vi "LPT-LIBS-Spectra Acquire.vi"(8 "error in":errorcluster, 9 "Exposure time [ms]":dbl=50.0 format="%#.6g", 10 "LIBS Dark Array":dbl[](array[numeric])) -> (0 "error out":errorcluster, 1 "Removed background":dbl[](graph), 2 "Raw Data":dbl[](graph), 3 "Spectrum":cluster{dbl[], dbl[]}(graph))   [LabVIEW 2019]
uses:
  <vilib>/Analysis/NI_AAL_SigProc.lvlib
panel:
  in  "threshold":dbl format="%0.2f"
  out "Locations":dbl[](array[numeric])
  out "Amplitudes":dbl[](array[numeric])
  out "# found":i32
  in  "polynomial order":i32=3
  in  "baseline (0)":dbl
  in  "RCF radius (25)":i32=60
  out "Filtered Spectrum":cluster{"Wavelengths":dbl[], "Filtered X":dbl[]}(graph)
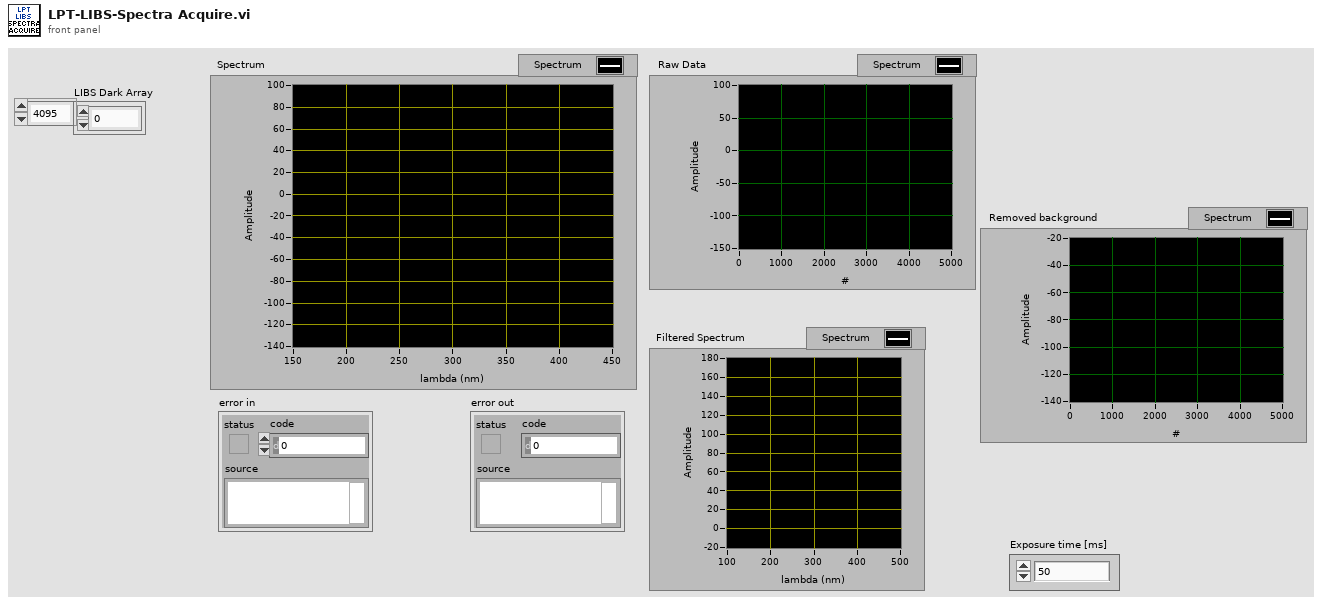
[diagram p1: front panel]
types:
  T1 = cluster{"Wavelength axis":dbl[], "Mean raw spectrum":dbl[]}
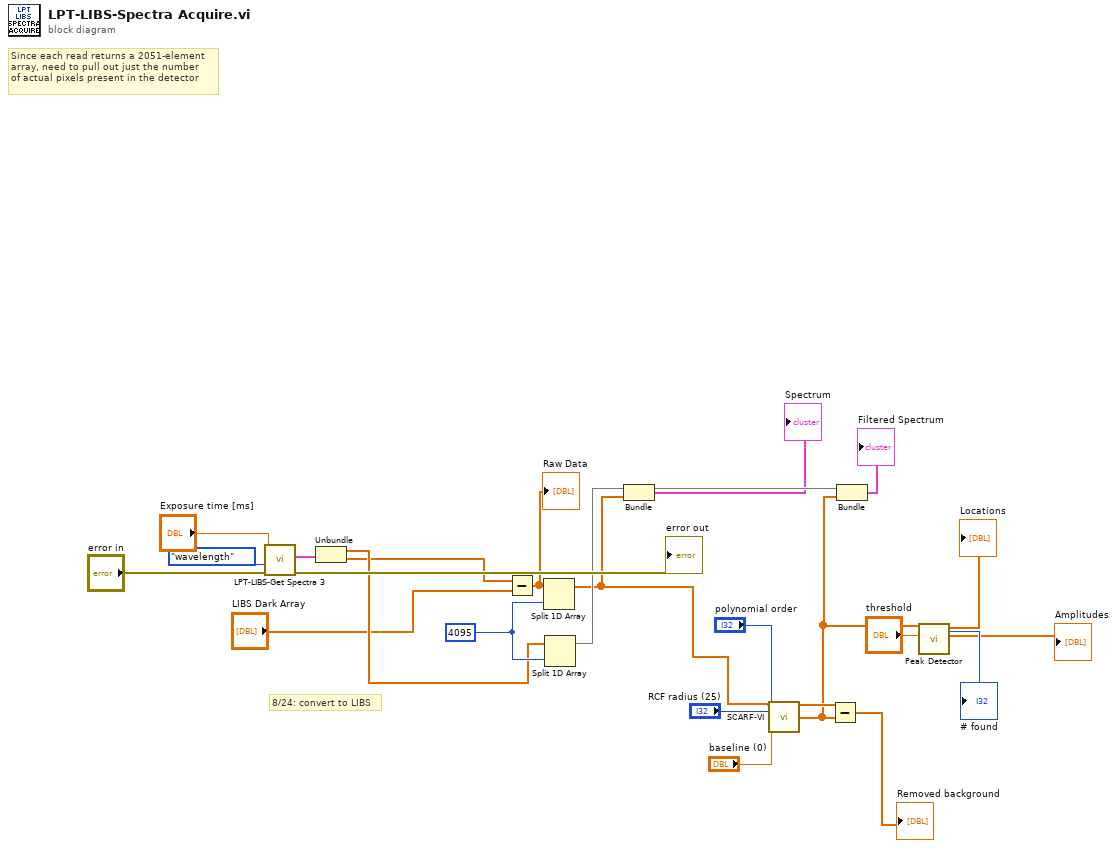
[diagram p0: block diagram]
diagram:
  w15 = 4095 ("index")
  # "8/24: convert to LIBS"
  # "Since each read returns a 2051-element\narray, need to pull out just the number\nof actual pixels present in the detector"
  n1 = call "LPT-LIBS-Get Spectra 3.vi"("error in"="error in", "x-axis representation:\npixels or wavelength?"=enum16{"wavelength", "pixels"}."wavelength" ("x-axis representation:\npixels or wavelength?"), "Exposure time [ms]"="Exposure time [ms]") -> ("error out"=→"error out":errorcluster, "Spectrum graph"=w2:T1)  [unwired: 7 in]
  n2 = Unbundle(w2) -> ("Wavelength axis"=w14:dbl[], "Mean raw spectrum"=w8:dbl[])
  n3 = Subtract(x=w8, y="LIBS Dark Array") -> (x-y=w7:dbl[])
  "Raw Data" <- w7
  n4 = Split 1D Array(array=w7, index=w15) -> (first subarray=w9:dbl[])  [unwired: 1 out]
  n5 = Split 1D Array(array=w14, index=w15) -> (first subarray=w11:dbl[])  [unwired: 1 out]
  n6 = Bundle(w11, w9) -> (→"Spectrum":cluster{dbl[], dbl[]})  [unwired: 1 in]
  n7 = call "SCARF-VI.vi"("input spectrum"=w9, "RCF radius (25)"="RCF radius (25)", "baseline (0)"="baseline (0)", "polynomial order"="polynomial order") -> ("bypassed spectrum"=w4:dbl[], "residue"=w3:dbl[])  [unwired: 7 in, 3 out]
  n8 = Subtract(x=w4, y=w3) -> (x-y=→"Removed background":dbl[])
  n9 = Bundle(w11, "residue"=w3) -> (→"Filtered Spectrum":cluster{dbl[], "residue":dbl[]})  [unwired: 1 in]
  n10 = call <vilib>:"Peak Detector.vi"("threshold"="threshold", "X"=w3) -> ("Amplitudes"=→"Amplitudes":dbl[], "Locations"=→"Locations":dbl[], "# found"=→"# found":i32)  [unwired: 5 in, 2 out]
